vi "LakeShore 372 Zones.vi"() -> ()   [LabVIEW 2021]
doc: "This VI manages the zones for the LakeShore Model 370 Temperature Controller. Set the address and run the VI. The current values are read and entered into the table. Add any additional values or edit the current values, you do not need to sort by temperature. When the OK button is pressed the values are sorted and uploaded. The indicators will tell you which zones have been updated.\n\nScott Hannahs, <sth@magnet.fsu.edu> NHMFL-FSU, May 2003"
panel:
  in  "Heater":bool
  out "Updated":bool[](array[boolean])
  in  "OK Button":bool
  in  "VISA Session":refnum<visa-resource-name>
  in  "Zone List":T1(array[cluster])=[{"Limit"=0.01, "P"=1.0, "I"=5.0, "D"=0.0, "Manual"=0.0, "Heater Range (0: Off)"=0.0, "Rate K/S"=0.0, "Relay Low (0: Off)"=0.0, "Relay High (0: Off)"=0.0}, {"Limit"=0.02, "P"=1.0, "I"=5.0, "D"=0.0, "Manual"=0.0, "Heater Range (0: Off)"=0.0, "Rate K/S"=0.0, "Relay Low (0: Off)"=0.0, "Relay High (0: Off)"=0.0}, {"Limit"=0.35, "P"=20.0, "I"=5.0, "D"=0.0, "Manual"=10.0, "Heater Range (0: Off)"=2.0, "Rate K/S"=0.0, "Relay Low (0: Off)"=0.0, "Relay High (0: Off)"=0.0}, {"Limit"=0.5, "P"=5.0, "I"=5.0, "D"=0.0, "Manual"=10.0, "Heater Range (0: Off)"=3.0, "Rate K/S"=0.0, "Relay Low (0: Off)"=0.0, "Relay High (0: Off)"=0.0}, {"Limit"=0.75, "P"=1.0, "I"=5.0, "D"=0.0, "Manual"=10.0, "Heater Range (0: Off)"=4.0, "Rate K/S"=0.0, "Relay Low (0: Off)"=0.0, "Relay High (0: Off)"=0.0}, {"Limit"=1.25, "P"=1.0, "I"=5.0, "D"=0.0, "Manual"=10.0, "Heater Range (0: Off)"=4.0, "Rate K/S"=0.0, "Relay Low (0: Off)"=0.0, "Relay High (0: Off)"=0.0}, {"Limit"=4.0, "P"=0.5, "I"=5.0, "D"=0.0, "Manual"=10.0, "Heater Range (0: Off)"=5.0, "Rate K/S"=0.0, "Relay Low (0: Off)"=0.0, "Relay High (0: Off)"=0.0}, {"Limit"=5.5, "P"=0.5, "I"=5.0, "D"=0.0, "Manual"=10.0, "Heater Range (0: Off)"=5.0, "Rate K/S"=0.0, "Relay Low (0: Off)"=0.0, "Relay High (0: Off)"=0.0}, {"Limit"=7.0, "P"=0.25, "I"=5.0, "D"=0.0, "Manual"=10.0, "Heater Range (0: Off)"=6.0, "Rate K/S"=0.0, "Relay Low (0: Off)"=0.0, "Relay High (0: Off)"=0.0}, {"Limit"=9.25, "P"=0.25, "I"=5.0, "D"=0.0, "Manual"=10.0, "Heater Range (0: Off)"=6.0, "Rate K/S"=0.0, "Relay Low (0: Off)"=0.0, "Relay High (0: Off)"=0.0}] {"Rate K/S" format="%.3g"; "Relay High (0: Off)" items=["Off", "On"]; "Relay Low (0: Off)" items=["Off", "On"]; "Heater Range (0: Off)" items=["Off", "31.6 uA", "100 uA", "316 uA", "1.00 mA", "3.16 mA", "10.0 mA", "31.6 mA", "100 mA"]; "Manual" format="%.1f"; "D" format="%.1f"; "I" format="%.1f"; "P" format="%.3f"; "Limit" format="%.3f"}
  # "The Limit starts at 0K and the limit is the upper limit for the zone.  The data can be entered in any order and will be sorted by the Limit value before it is sent to the LakeShore 370."
  # "Warmup"
  # "Sample"
  # "Relay\n#1  #2"
  # "Zone #"
  # "Rate K/min"
  # "Limit (K)"
  # "P"
  # "I (sec)"
  # "D (sec)"
  # "Manual"
  # "Range"
  # "1"
  # "2"
  # "3"
  # "4"
  # "5"
  # "6"
  # "7"
  # "8"
  # "9"
  # "10"
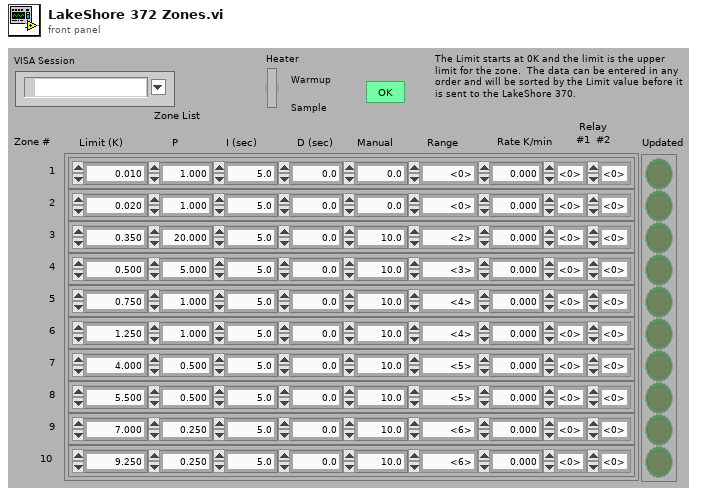
[diagram p1: front panel]
types:
  T1 = cluster{"Limit":dbl, "P":dbl, "I":dbl, "D":dbl, "Manual":dbl, "Heater Range (0: Off)":dbl, "Rate K/S":dbl, "Relay Low (0: Off)":dbl, "Relay High (0: Off)":dbl}[]
  T2 = cluster{"Measurement[0]":dbl, "Measurement[1]":dbl, "Measurement[2]":dbl, "Measurement[3]":dbl, "Measurement[4]":dbl, "Measurement[5]":dbl, "Measurement[6]":dbl, "Measurement[7]":dbl, "Measurement[8]":dbl}
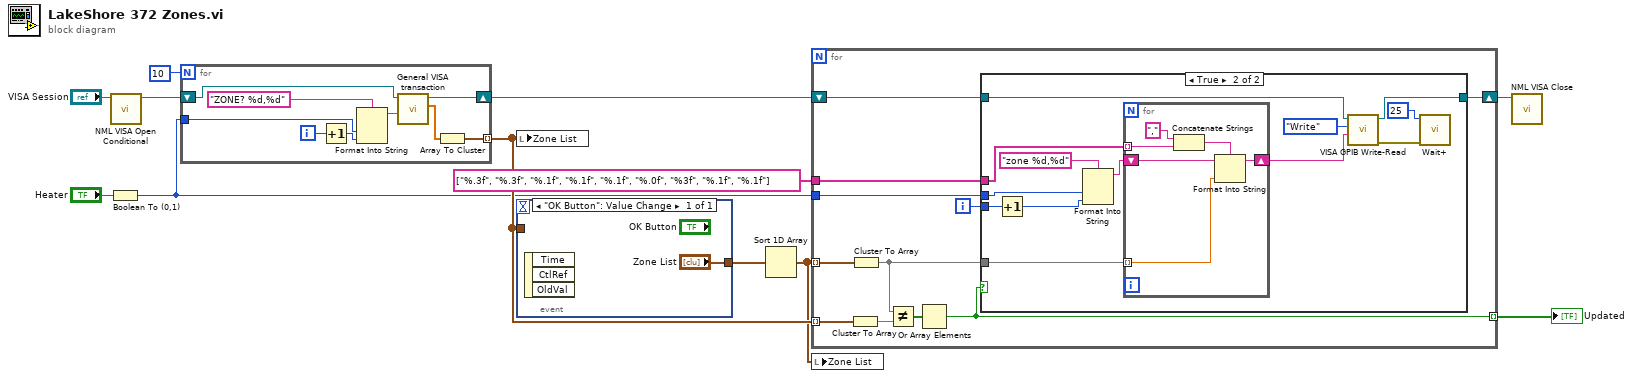
[diagram p0: block diagram]
diagram:
  n1 = Boolean To (0,1)(Boolean="Heater") -> (0, 1=w1:i16)
  n2 = call "NML VISA Open Conditional.vi"("VISA resource name"="VISA Session") -> ("dup VISA Session"=w4:refnum<visa-resource-name>)  [unwired: 8 in, 2 out]
  n3 = for {
    N: 10 -> [_]
    tunnel: [w16] -> w8 mode=indexing
    shift-right: [w15] -> w5
    shift-left: w4 -> [w18]
    tunnel: w1 -> [w13]
    i -> [w21]
    n4 = Increment(x=w21) -> (x+1=w14:i32)
    n5 = Format Into String(format string="ZONE? %d,%d", w13, w14) -> (resulting string=w19:string)  [unwired: 2 in, 1 out]
    n6 = call "General VISA transaction.vi"("Command String"=w19, "VISA Session"=w18) -> ("Measurement"=w17:dbl[], "dup VISA Session"=w15:refnum<visa-resource-name>)  [unwired: 4 in, 4 out]
    n7 = Array To Cluster(array=w17) -> (cluster=w16:T2)
  }
  n8 = local write "Zone List"(w8) -> ()
  n9 = event shown="[0] \"OK Button\": Value Change" {
    selector: _ -> [_]
    dyn-events: _ -> [_]
    timeout: _ -> [_]
    tunnel: ["Zone List"] -> w10
    tunnel: w8 -> [_]
    event "OK Button": Value Change {
      n10 = event-data() -> ()  [unwired: 1 in, 3 out]
    }
  }
  n11 = Sort 1D Array(array=w10) -> (sorted array=w6:T1)
  n12 = for {
    tunnel: w6 -> [w33] mode=indexing
    tunnel: string[] ["%.3f", "%.3f", "%.1f", "%.1f", "%.1f", "%.0f", "%3f", "%.1f", "%.1f"] -> [w30]
    tunnel: w8 -> [w29] mode=indexing
    tunnel: [w26] -> w7 mode=indexing
    shift-right: [w24] -> w3
    shift-left: w5 -> [w25]
    tunnel: w1 -> [w23]
    i -> [w31]
    n13 = Cluster To Array(cluster=w29) -> (array=w28:dbl[])
    n14 = Cluster To Array(cluster=w33) -> (array=w32:dbl[])
    n15 = Not Equal?(x=w32, y=w28) -> (x != y?=w27:bool[])
    n16 = Or Array Elements(Boolean array=w27) -> (logical OR=w26:bool)
    n17 = case shown="True" w26 {
      tunnel: w32 -> [_ w47]
      tunnel: w31 -> [_ w46]
      tunnel: w30 -> [_ w43]
      tunnel: w25 -> [w34 w38]
      tunnel: [w34 w37] -> w24
      tunnel: w23 -> [_ w35]
      frame False {
      }
      frame True {
        n18 = Increment(x=w46) -> (x+1=w36:i32)
        n19 = Format Into String(format string="zone %d,%d", w35, w36) -> (resulting string=w44:string)  [unwired: 2 in, 1 out]
        n20 = for {
          tunnel: w47 -> [w52] mode=indexing
          shift-right: [w51] -> w42
          shift-left: w44 -> [w53]
          tunnel: w43 -> [w49] mode=indexing
          n21 = Concatenate Strings("," ("string"), w49) -> (w50:string)
          n22 = Format Into String(format string=w50, initial string=w53, w52) -> (resulting string=w51:string)  [unwired: 1 in, 1 out]
        }
        n23 = call "VISA GPIB Write-Read.vi"("Command"=w42, "Action"=enum16{"Write", "Read", "Write & Read"}."Write", "VISA resource name"=w38) -> ("error out"=w40:errorcluster, "dup VISA Session"=w37:refnum<visa-resource-name>)  [unwired: 5 in, 2 out]
        n24 = call "Wait+.vi"("Error In"=w40, "milliseconds to wait"=u32 25) -> ()  [unwired: 4 in, 2 out]
      }
    }
  }
  "Updated" <- w7
  n25 = local write "Zone List"(w6) -> ()
  n26 = call "NML VISA Close.vi"("VISA resource name"=w3) -> ()  [unwired: 10 in, 1 out]
